vi "Fire User Event - Next State.vi"(8 "Error In":errorcluster, 10 "\"UI Handler loop\" case to execute":T1) -> (0 "Error Out":errorcluster)   [LabVIEW 2020]
doc: "Send the Stop event to stop the Event Handling Loop."
uses:
  Typedefs/Top level VI states.ctl
  Typedefs/Set Main VI cursor.ctl
  Global Variables/gl_User Events.vi
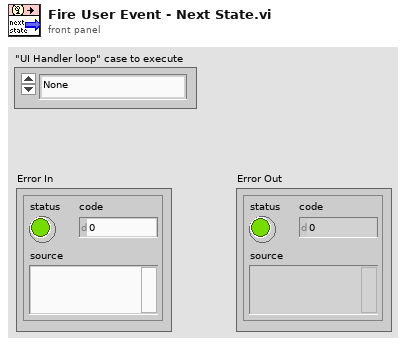
[diagram p1: front panel]
types:
  T1 = typedef "Top level VI states.ctl" = enum16{"None", "Initialise UI", "<STACK PROTOCOL STATES>", "AOL Zstack-START", "AOL Zstack-STOP", "Motor Zstack-START", "Motor Zstack-STOP", "<ACQUISITION PROTOCOL STATES> ", "Functional Acquisition-START", "Functional Acquisition-STOP", "Single Plane Acquisition-START", "Single Plane Acquisition-STOP", "Volume Acquisition-START", "Volume Acquisition-STOP", "<LIVE IMAGING PROTOCOL STATES>", "Live Imaging-START", "Live Imaging-STOP", "Live Plane Imaging-START", "Live Plane Imaging-STOP", "Live Volume Imaging-START", "Live Volume Imaging-STOP", "<MOVEMENT CORRECTION PROTOCOL STATES>", "EXIT"}
  T2 = typedef "Set Main VI cursor.ctl" = enum16{"Release busy cursor", "Set busy cursor"}
  T3 = cluster{"User Event - Stop":refnum<user-event>, "User Event - Next State":refnum<user-event>}
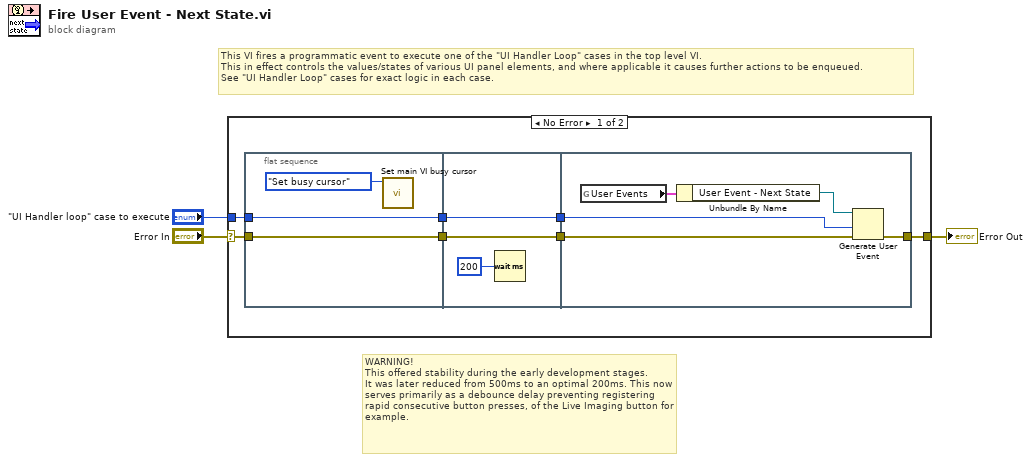
[diagram p0: block diagram]
diagram:
  # "WARNING!\nThis offered stability during the early development stages.\nIt was later reduced from 500ms to an optimal 200ms. This now serves primarily as a debounce delay preventing registering rapid consecutive button presses, of the Live Imaging button for example."
  # "This VI fires a programmatic event to execute one of the \"UI Handler Loop\" cases in the top level VI.\nThis in effect controls the values/states of various UI panel elements, and where applicable it causes further actions to be enqueued.\nSee \"UI Handler Loop\" cases for exact logic in each case."
  n1 = case shown="No Error" "Error In" {
    selector: "Error In" -> [w9 w22]
    tunnel: [w10 w22] -> w2
    tunnel: "\"UI Handler loop\" case to execute" -> [w8 _]
    frame No Error {
      n2 = flat-sequence {
        tunnel: w8 -> [w12]
        tunnel: w9 -> [w13]
        tunnel: [w13] -> w5
        tunnel: [w12] -> w4
        tunnel: [w16] -> w7
        tunnel: [w15] -> w6
        tunnel: w5 -> [w16]
        tunnel: w4 -> [w15]
        tunnel: [w21] -> w10
        tunnel: w7 -> [w20]
        tunnel: w6 -> [w17]
        frame #0 {
          n3 = call "Set main VI busy cursor.vi"("Main VI's cursor"=Set_Main_VI_cursor."Set busy cursor") -> ()  [unwired: 10 in, 1 out]
        }
        frame #1 {
          n4 = Wait (ms)(milliseconds to wait=u32 200) -> ()  [unwired: 1 out]
        }
        frame #2 {
          n5 = global read "gl_User Events.vi" "User Events"() -> (w19:T3)
          n6 = Unbundle By Name(w19) -> ("User Event - Next State"=w18:refnum<user-event>)
          n7 = Generate User Event(user event=w18, event data cluster=w17, error in=w20) -> (error out=w21:errorcluster)  [unwired: 1 in, 1 out]
        }
      }
    }
    frame Error {
    }
  }
  "Error Out" <- w2
